vi "List All Trees Priv.vi"(8 "error in":errorcluster, 11 "Tree Dict":variant) -> (0 "error out":errorcluster, 1 "Tree Names":string[](array[string]), 2 "Tree IDs":string[](array[string]), 3 "Tree Dict":variant)   [LabVIEW 2017, in "Tree API.lvlib" / "Tree.lvclass"]
uses:
  Tree.lvclass
  Typedefs/Tree Cluster.ctl
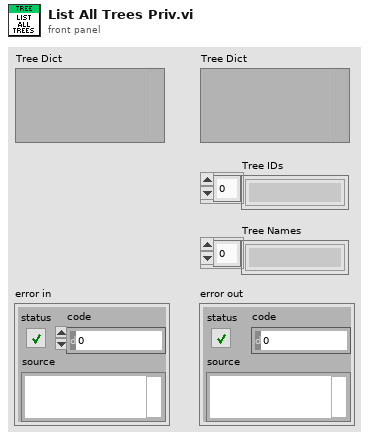
[diagram p1: front panel]
types:
  T1 = typedef "Tree API.lvlib/Tree.lvclass/Tree Cluster.ctl" = cluster{"Unique ID":string, "Parent ID":string, "Child IDs":string[], "Name":string, "MetaData":string, "Data IDs":string[]}
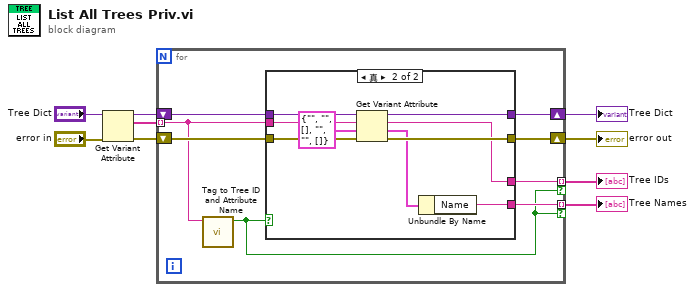
[diagram p0: block diagram]
diagram:
  n1 = Get Variant Attribute(Variant="Tree Dict", error in="error in") -> (duplicate Variant=w6:variant, names=w3:string[], error out=w5:errorcluster)  [unwired: 2 in, 1 out]
  n2 = for {
    tunnel: w3 -> [w15] mode=indexing
    tunnel: [w11] -> w4 mode=indexing if=w10
    shift-right: [w14] -> w7
    shift-left: w6 -> [w17]
    shift-right: [w13] -> w8
    shift-left: w5 -> [w16]
    tunnel: [w12] -> w9 mode=indexing if=w10
    n3 = call "Tag to Tree ID and Attribute Name.vi"("Tag"=w15) -> ("Tree"=w10:bool)  [unwired: 8 in, 2 out]
    n4 = case shown="真" w10 {
      tunnel: w17 -> [w19 w27]
      tunnel: w16 -> [w18 w26]
      tunnel: w15 -> [_ w20]
      tunnel: [w19 w24] -> w14
      tunnel: [w18 w23] -> w13
      tunnel: [_ w21] -> w12
      tunnel: [_ w20] -> w11
      frame False {
      }
      frame True {
        n5 = Get Variant Attribute(Variant=w27, name=w20, default value (empty Variant)=T1 {"Unique ID"="", "Parent ID"="", "Child IDs"=[], "Name"="", "MetaData"="", "Data IDs"=[]} ("Cluster of class private data"), error in=w26) -> (duplicate Variant=w24:variant, value=w22:T1, error out=w23:errorcluster)  [unwired: 1 out]
        n6 = Unbundle By Name(w22) -> ("Name"=w21:string)
      }
    }
  }
  "Tree Names" <- w9
  "error out" <- w8
  "Tree Dict" <- w7
  "Tree IDs" <- w4
